vi "Mem1024_Fast3.vi"(6 "Reset":bool, 8 "Init":bool, 9 "Phi2":bool, 10 "Phi1":bool, 11 "In":bool) -> (0 "Mem":bool[](array[boolean]), 3 "Out":bool)   [LabVIEW 2012]
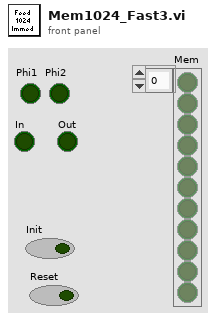
[diagram p1: front panel]
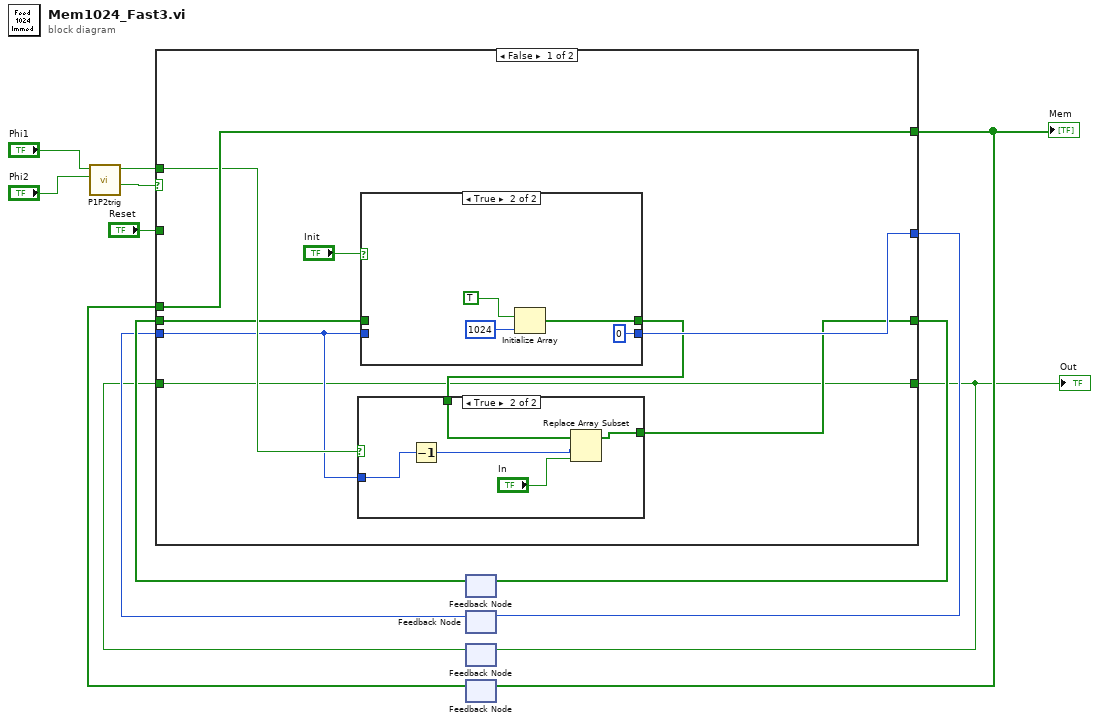
[diagram p0: block diagram]
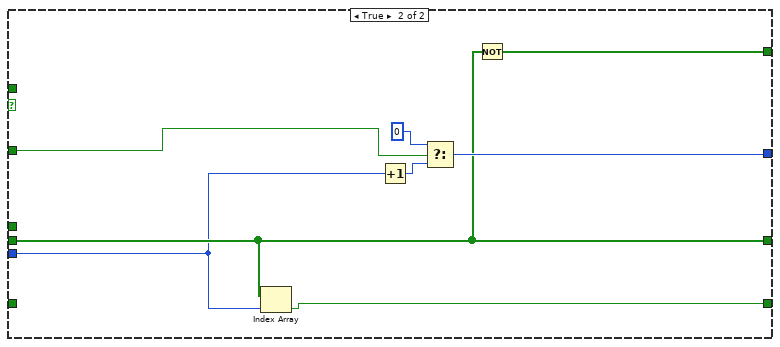
[diagram p4: hidden frame]
diagram:
  n1 = call "P1P2trig.vi"("Phi2"="Phi2", "Phi1"="Phi1") -> ("TrigUp"=w11:bool, "TrigDown"=w1:bool)  [unwired: 7 in, 1 out]
  n2 = feedback #1() -> (w10:bool[])  [unwired: 1 in]
  n3 = feedback #2() -> (w8:i32)  [unwired: 1 in]
  n4 = feedback #3() -> (w6:bool)  [unwired: 1 in]
  n5 = feedback #4() -> (w4:bool[])  [unwired: 1 in]
  n6 = case shown="False" w11 {
    tunnel: w10 -> [w18 w37]
    tunnel: [w15 w37] -> w9
    tunnel: [w14 w38] -> w2
    tunnel: w8 -> [w17 w36]
    tunnel: [w21 w40] -> w7
    tunnel: w6 -> [w14 _]
    tunnel: [w20 w35] -> w5
    tunnel: w4 -> [w20 _]
    tunnel: "Reset" -> [_ w39]
    tunnel: w1 -> [w19 _]
    frame False {
      n7 = case shown="True" "Init" {
        tunnel: [w30 w32] -> w16
        tunnel: w18 -> [w30 _]
        tunnel: w17 -> [w29 _]
        tunnel: [w29 0 ("y")] -> w21
        frame False {
        }
        frame True {
          n8 = Initialize Array(TRUE, 1024 ("dimension size")) -> (w32:bool[])
        }
      }
      n9 = case shown="True" w19 {
        tunnel: [w23 w26] -> w15
        tunnel: w16 -> [w23 w25]
        tunnel: w17 -> [_ w28]
        frame False {
        }
        frame True {
          n10 = Decrement(x=w28) -> (x-1=w24:i32)
          n11 = Replace Array Subset(array=w25, new element="In", index=w24) -> (w26:bool[])
        }
      }
    }
    frame True {
      n12 = Index Array(array=w37, index=w36) -> (element=w38:bool)
      n13 = Increment(x=w36) -> (x+1=w41:i32)
      n14 = Select(t=0 ("y"), s=w39, f=w41) -> (s? t:f=w40:i32)
      n15 = Not(x=w37) -> (.not. x?=w35:bool[])
    }
  }
  "Out" <- w2
  "Mem" <- w5
  n16 = feedback-in #1(w9) -> ()
  n17 = feedback-in #2(w7) -> ()
  n18 = feedback-in #3(w2) -> ()
  n19 = feedback-in #4(w5) -> ()
